vi "RP100.VISA RW.vi"(8 "error in (no error)":errorcluster, 10 "Write":string, 11 "VISA Refnum in":refnum<visa-resource-name>) -> (0 "error out":errorcluster, 2 "Read":string, 3 "VISA Refnum out":refnum<visa-resource-name>)   [LabVIEW 2019, in "RP100.lvclass"]
uses:
  RP100.lvclass
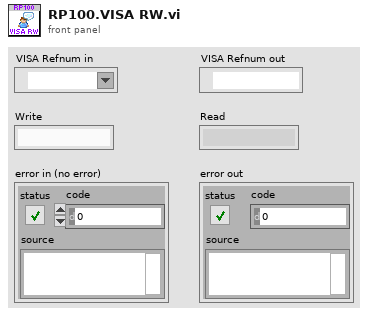
[diagram p1: front panel]
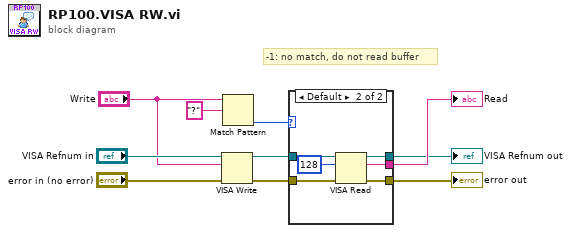
[diagram p0: block diagram]
diagram:
  # "-1: no match, do not read buffer"
  n1 = VISA Write(VISA resource name="VISA Refnum in", write buffer="Write", error in (no error)="error in (no error)") -> (VISA resource name out=w2:refnum<visa-resource-name>, error out=w3:errorcluster)  [unwired: 1 out]
  n2 = Match Pattern(string="Write", regular expression="?") -> (offset past match=w1:i32)  [unwired: 1 in, 3 out]
  n3 = case shown="Default" w1 {
    tunnel: [_ w18] -> w9
    tunnel: [w11 w17] -> w8
    tunnel: [w12 w16] -> w6
    tunnel: w3 -> [w11 w15]
    tunnel: w2 -> [w12 w14]
    frame -1 {
    }
    frame Default {
      n4 = VISA Read(VISA resource name=w14, byte count=u32 128, error in (no error)=w15) -> (VISA resource name out=w16:refnum<visa-resource-name>, read buffer=w18:string, error out=w17:errorcluster)  [unwired: 1 out]
    }
  }
  "Read" <- w9
  "error out" <- w8
  "VISA Refnum out" <- w6
